vi "Transmitter_Example.vi"() -> ()   [LabVIEW 2018]
uses:
  <vilib>/picture/picture.llb/imagedata.ctl
  <instrlib>/niUSRP/niUSRP Write Tx Data (CDB Cluster).vi
panel:
  in  "Numeric":i32
  out "new picture":picture
  out "image data":T1
  in  "path to BMP file":path
  in  "Modulation parameter":T2
  out "Bits length":i32
  out "Frame Duration":dbl format="%#_6p"
  out "Waveform Graph":cluster{"t0":dbl, "dt":dbl, "Y":dbl[]}(graph)
  in  "stop":bool
  in  "String":string="PENS"
  out "USRP CoercedParamters":T3={"coerced IQ rate"=100000.0, "coerced carrier frequency"=100000.0, "coerced gain"=0.0} {"coerced gain" format="%#_6f"; "coerced carrier frequency" format="%#_6p"; "coerced IQ rate" format="%#_6p"}
  out "error out":errorcluster
  in  "error in (no error)":errorcluster
  in  "USRP ControledParameters":T4={"active antenna"="TX1", "gain"=0.0, "carrier frequency"=915000000.0, "IQ rate"=1000000.0} {"IQ rate" format="%#_6p"; "carrier frequency" format="%#_6p"; "gain" format="%#_6f"}
  in  "device names":refnum<k15>="192.168.10.1"
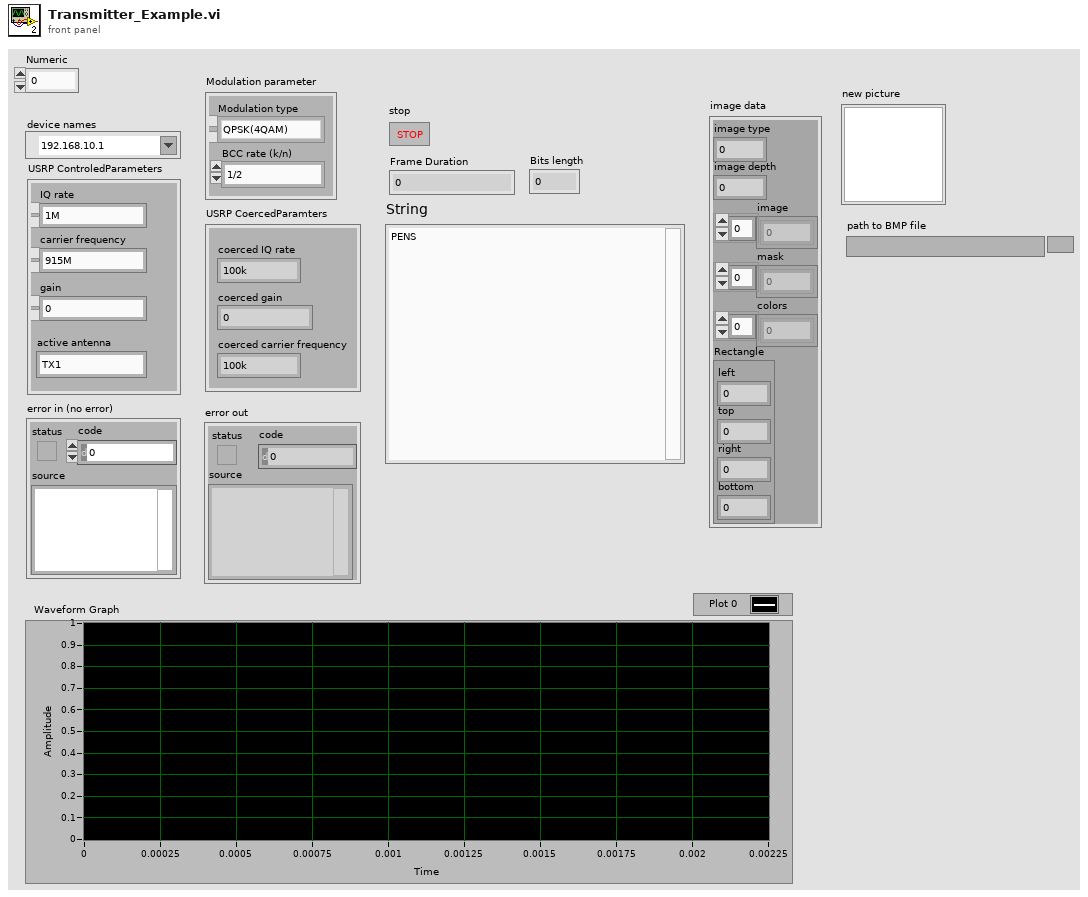
[diagram p1: front panel]
types:
  T1 = typedef "imagedata.ctl" = cluster{"image type":i32, "image depth":i32, "image":u8[], "mask":u8[], "colors":u32[], "Rectangle":cluster{"left":i16, "top":i16, "right":i16, "bottom":i16}}
  T2 = cluster{"Modulation type":enum16{"QPSK(4QAM)", "64QAM", "16QAM", "BPSK"}, "BCC rate (k/n)":enum16{"1/2", "2/3", "3/4"}}
  T3 = cluster{"coerced IQ rate":dbl, "coerced carrier frequency":dbl, "coerced gain":dbl}
  T4 = cluster{"active antenna":string, "gain":dbl, "carrier frequency":dbl, "IQ rate":dbl}
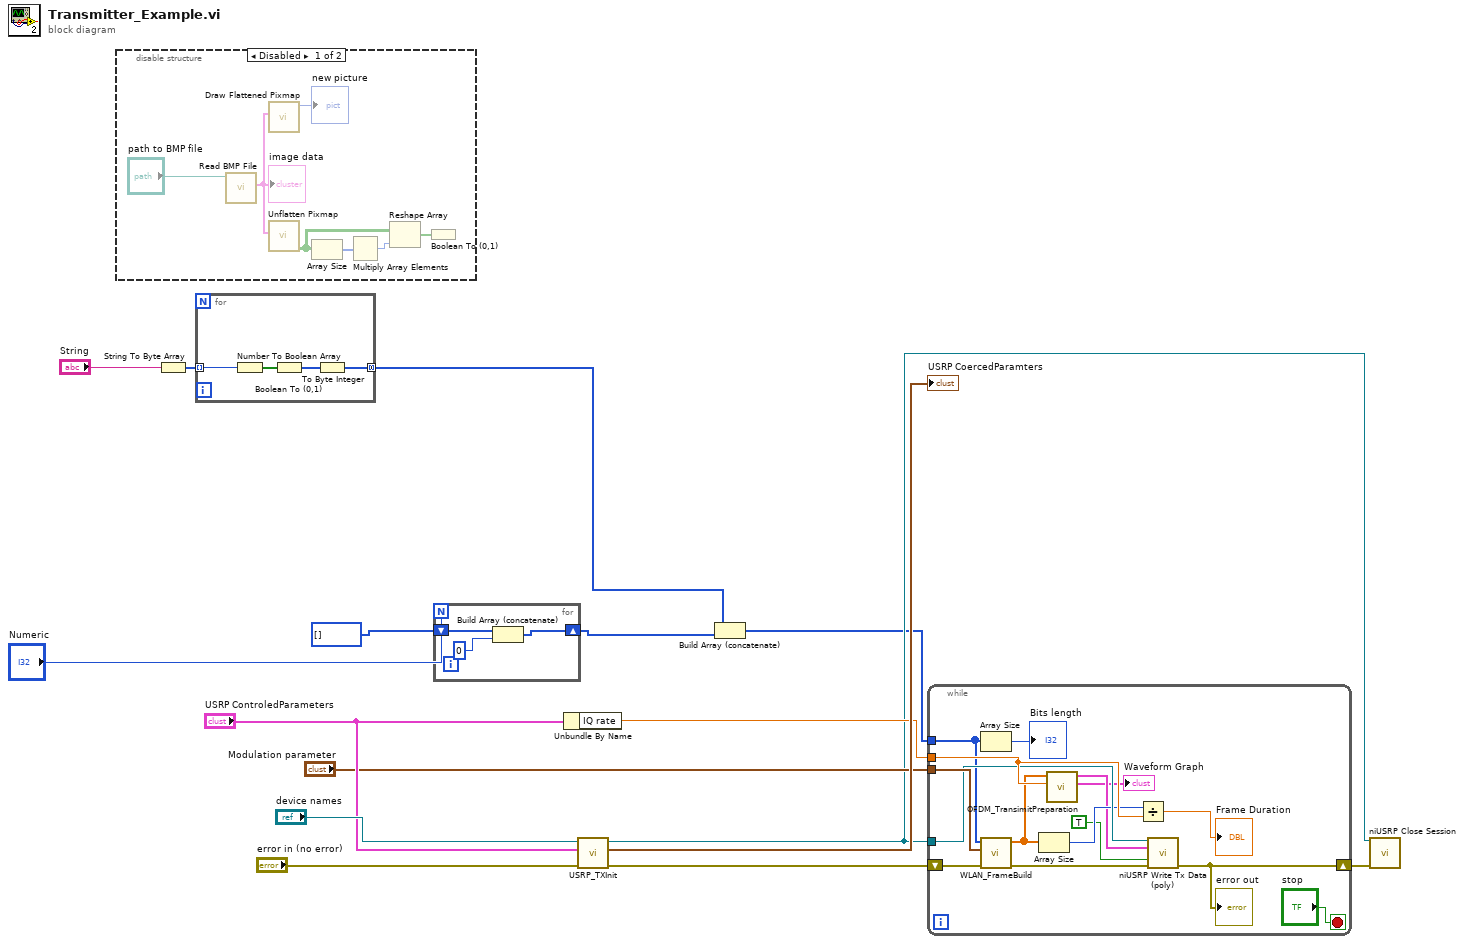
[diagram p0: block diagram]
diagram:
  n1 = disable-structure shown="Disabled" {
    frame Disabled {
      n2 = call <vilib>:"Read BMP File.vi"("path to BMP file"="path to BMP file") -> ("image data"=w21:T1)  [unwired: 8 in, 2 out]
      "image data" <- w21
      n3 = call <vilib>:"Draw Flattened Pixmap.vi"("image data"=w21) -> ("new picture"=→"new picture":picture)  [unwired: 8 in]
      n4 = call <vilib>:"Unflatten Pixmap.vi"("image data"=w21) -> ("1-bit pixmap"=w19:bool[][])  [unwired: 4 in, 6 out]
      n5 = Array Size(array=w19) -> (size(s)=w20:i32[])
      n6 = Multiply Array Elements(1:w20) -> (0:w18:i32)
      n7 = Reshape Array(w19, w18) -> (w17:bool[])
      n8 = Boolean To (0,1)(Boolean=w17) -> ()  [unwired: 1 out]
    }
    frame Enabled {
    }
  }
  n9 = String To Byte Array(string="String") -> (unsigned byte array=w7:u8[])
  n10 = for {
    tunnel: w7 -> [w27] mode=indexing
    tunnel: [w24] -> w3 mode=concatenating
    n11 = Number To Boolean Array(number=w27) -> (Boolean array=w26:bool[])
    n12 = Boolean To (0,1)(Boolean=w26) -> (0, 1=w25:i16[])
    n13 = To Byte Integer(number=w25) -> (8bit integer=w24:i8[])
  }
  n14 = for {
    N: "Numeric" -> [_]
    shift-right: [w28] -> w2
    shift-left: i32[] [] -> [w30]
    n15 = Build Array (concatenate)(w30, 0) -> (w28:i32[])
  }
  n16 = Unbundle By Name("USRP ControledParameters") -> ("IQ rate"=w10:dbl)
  n17 = call "USRP_TXInit.vi"("device names"="device names", "USRP ControledParameters"="USRP ControledParameters", "error in (no error)"="error in (no error)") -> ("session handle out"=w9:refnum<k15>, "USRP CoercedParamters"=→"USRP CoercedParamters":T3, "error out"=w11:errorcluster)  [unwired: 5 in]
  n18 = Build Array (concatenate)(w3, w2) -> (w1:i32[])
  n19 = while {
    tunnel: "Modulation parameter" -> [w45]
    tunnel: w10 -> [w43]
    tunnel: w9 -> [w42]
    tunnel: w1 -> [w40]
    shift-right: [w41] -> w8
    shift-left: w11 -> [w44]
    stop <- "stop" stop-if-true
    n20 = Array Size(array=w40) -> (size(s)=→"Bits length":i32)
    n21 = call "WLAN_FrameBuild.vi"("error in (no error)"=w44, "Modulation parameter"=w45, "data in"=w40) -> ("error out"=w35:errorcluster, "output array"=w34:cdb[])  [unwired: 5 in, 2 out]
    n22 = Array Size(array=w34) -> (size(s)=w39:i32)
    n23 = call "OFDM_TransimitPreparation.vi"("IQ rate"=w43, "array"=w34) -> ("output cluster 2"=→"Waveform Graph":cluster{"t0":dbl, "dt":dbl, "Y":cdb[]}, "output cluster"=w37:cluster{"t0":dbl, "dt":dbl, "Y":cdb[]})  [unwired: 8 in]
    n24 = Divide(x=w39, y=w43) -> (x/y=→"Frame Duration":dbl)
    n25 = call-poly <instrlib>:"niUSRP Write Tx Data (poly).vi"("session handle"=w42, "data"=w37, "end of data?"=TRUE, "error in (no error)"=w35) -> ("error out"=w41:errorcluster)  [unwired: 10 in, 1 out]
    "error out" <- w41
  }
  n26 = call <instrlib>:"niUSRP Close Session.vi"("session handle"=w9, "error in (no error)"=w8) -> ()  [unwired: 13 in, 1 out]
